vi "Write State DVR.vi"(8 "error in (no error)":errorcluster, 10 "State DVR":refnum<data-value>, 11 "Stabilize Laser in":refnum<class "Stabilize Laser.lvclass">) -> (0 "error out":errorcluster, 3 "Stabilize Laser out":refnum<class "Stabilize Laser.lvclass">)   [LabVIEW 2013, in "Stabilize Laser.lvclass"]
uses:
  Stabilize Laser.lvclass
  Data/cPAS Data.lvclass
  Stabilize Laser.lvclass/Stabilize Laser.ctl
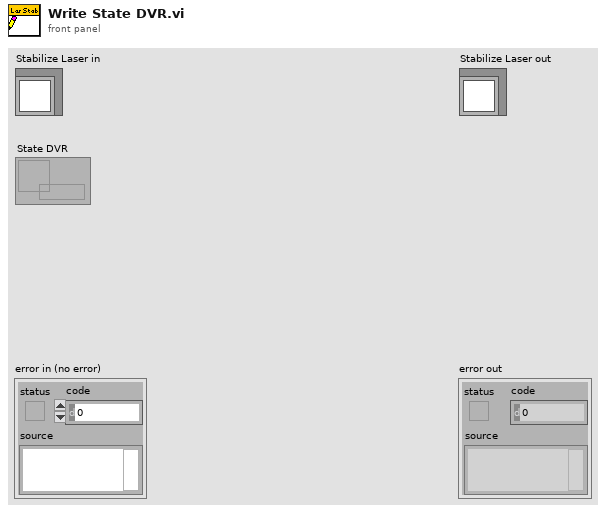
[diagram p1: front panel]
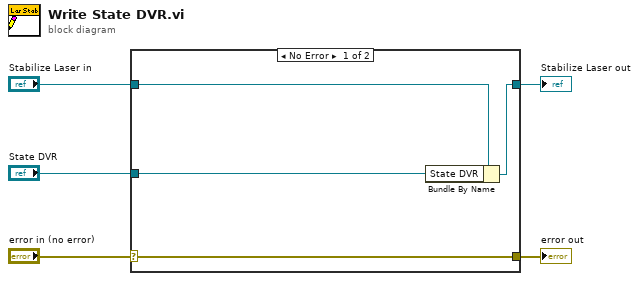
[diagram p0: block diagram]
diagram:
  n1 = case shown="No Error" "error in (no error)" {
    selector: "error in (no error)" -> [w9 w10]
    tunnel: [w9 w10] -> w4
    tunnel: [w7 w11] -> w2
    tunnel: "Stabilize Laser in" -> [w8 w11]
    tunnel: "State DVR" -> [w6 _]
    frame No Error {
      n2 = Bundle By Name(cluster=w8, "State DVR"=w6) -> (w7:refnum<class "Stabilize Laser.lvclass">)
    }
    frame Error {
    }
  }
  "error out" <- w4
  "Stabilize Laser out" <- w2
